vi "4155C Transfer-FPP v2.0.vi"(0 "VISA resource name in":refnum<visa-resource-name>="GPIB0::14::INSTR", 1 "FPP - Source":u32(ring) items=["VSU1  ", "VSU2  "], 2 "Gate":T4={"Gate Start"=0.0, "Gate Stop"=2.0, "Gate Step (linear only)"=1.0, "Gate Compliance"=0.0001, "Gate PComp"=0.0, "Range mode"=0, "Range"=6} {"Range" max=11 scale=0.0..11.0; "Range mode" items=["Auto", "Limited", "Fixed"]; "Gate PComp" min=0.0 max=2.0 format="%^.2e"; "Gate Compliance" min=0.0 max=0.1 format="%^.2e"; "Gate Step (linear only)" min=-100.0 max=100.0 format="%^.4e"; "Gate Stop" min=-100.0 max=100.0 format="%^.4e"; "Gate Start" min=-100.0 max=100.0 format="%^.4e"}, 3 "Drain":T5={"Drain Start"=0.0, "Drain Stop"=2.0, "Drain Compliance"=0.0001, "Drain Step"=1.0, "Drain PComp"=0.0, "Range mode"=0, "Range"=6} {"Range" max=11 scale=0.0..11.0; "Range mode" items=["Auto", "Limited", "Fixed"]; "Drain PComp" min=0.0 max=2.0 format="%^.2e"; "Drain Step" min=-100.0 max=100.0 format="%^.4e"; "Drain Compliance" min=0.0 max=0.1 format="%^.2e"; "Drain Stop" min=-100.0 max=100.0 format="%^.4e"; "Drain Start" min=-100.0 max=100.0 format="%^.4e"}, 4 "FPP - Drain":u32(ring)=1 items=["SMU1  ", "SMU2  ", "SMU3  ", "SMU4  ", "SMU5  ", "SMU6  "], 5 "Timings":T3={"integration time"=0, "Short/Long integration time"=0.00064, "hold time (sec)"=0.0, "delay time (sec)"=0.0, "Step Time (0 disables)"=0.0, "sweep method"=0, "Pulse period"=0.005, "Base voltage"=0.0, "Pulse width"=0.0005} {"Pulse width" min=0.0005 max=0.1 step=0.0001 format="%.4f"; "Base voltage" min=-100.0 max=100.0 format="%^.4e"; "Pulse period" min=0.005 max=1.0 step=0.0001 format="%.4f"; "sweep method" items=["Continuous", "Pulsed"]; "Step Time (0 disables)" min=0.0 format="%.2f"; "delay time (sec)" min=0.0 format="%.4f"; "hold time (sec)" min=0.0 format="%.4f"; "Short/Long integration time" min=0.0 format="%^.0e"; "integration time" scale=0.0..2.0}, 6 "error in (no error)":errorcluster, 8 "FPP - Gate":u32(ring)=2 items=["SMU1  ", "SMU2  ", "SMU3  ", "SMU4  ", "SMU5  ", "SMU6  "], 9 "FPP - Probe 1":u32(ring) items=["SMU1  ", "SMU2  ", "SMU3  ", "SMU4  ", "SMU5  ", "SMU6  "], 10 "sweep mode":u16(ring) items=["Single", "Double"], 11 "FPP - Probe 2":u32(ring)=3 items=["SMU1  ", "SMU2  ", "SMU3  ", "SMU4  ", "SMU5  ", "SMU6  "], 12 "Panel Controls":T2={"Emergency Stop"=refnum, "TransGraph Max"=1e-05, "Text/Graph (text=false)"=FALSE} {"TransGraph Max" format="%.2e"}) -> (16 "VG":dbl[](array[numeric]) format="%.2f", 17 "Outparams":T1={"V2 Start"=0.0, "V2 Step"=0.0, "Number of points"=1} {"V2 Step" format="%.2f"; "V2 Start" format="%^.4e"}, 20 "VISA Resource Name out":refnum<visa-resource-name>, 21 "Vprobe2":dbl[](array[numeric]) format="%.2f", 22 "ID":dbl[](array[numeric]) format="%.2f", 23 "IG":dbl[](array[numeric]) format="%.2f", 25 "Vprobe1":dbl[](array[numeric]) format="%.2f", 26 "error out":errorcluster)   [LabVIEW 2016]
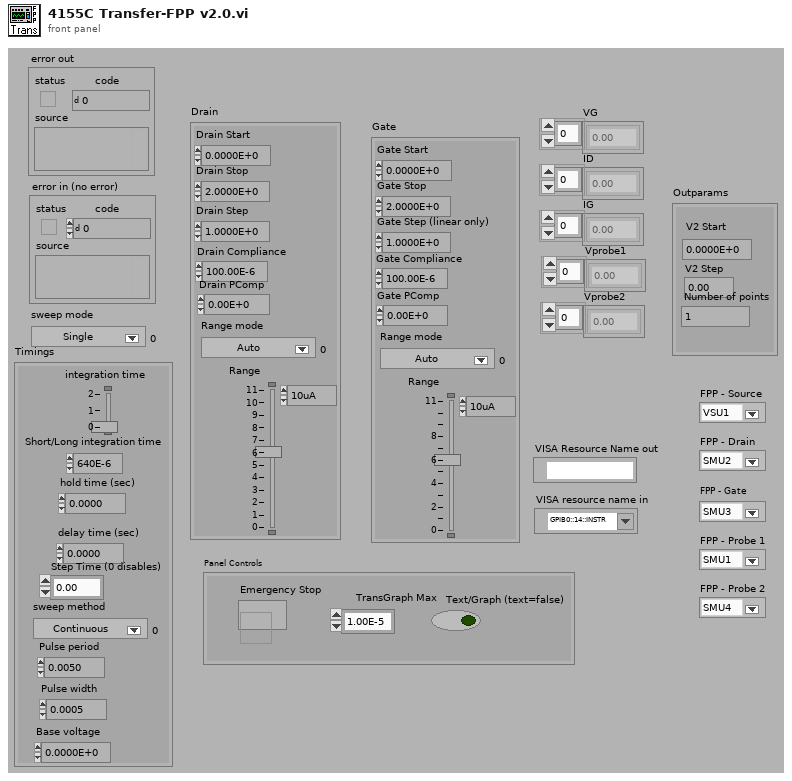
[diagram p1: front panel]
types:
  T1 = cluster{"V2 Start":dbl, "V2 Step":dbl, "Number of points":i32}
  T2 = cluster{"Emergency Stop":refnum<vi>, "TransGraph Max":dbl, "Text/Graph (text=false)":bool}
  T3 = cluster{"integration time":u32, "Short/Long integration time":dbl, "hold time (sec)":dbl, "delay time (sec)":dbl, "Step Time (0 disables)":dbl, "sweep method":u16, "Pulse period":dbl, "Base voltage":dbl, "Pulse width":dbl}
  T4 = cluster{"Gate Start":dbl, "Gate Stop":dbl, "Gate Step (linear only)":dbl, "Gate Compliance":dbl, "Gate PComp":dbl, "Range mode":u16, "Range":u8}
  T5 = cluster{"Drain Start":dbl, "Drain Stop":dbl, "Drain Compliance":dbl, "Drain Step":dbl, "Drain PComp":dbl, "Range mode":u16, "Range":u8}
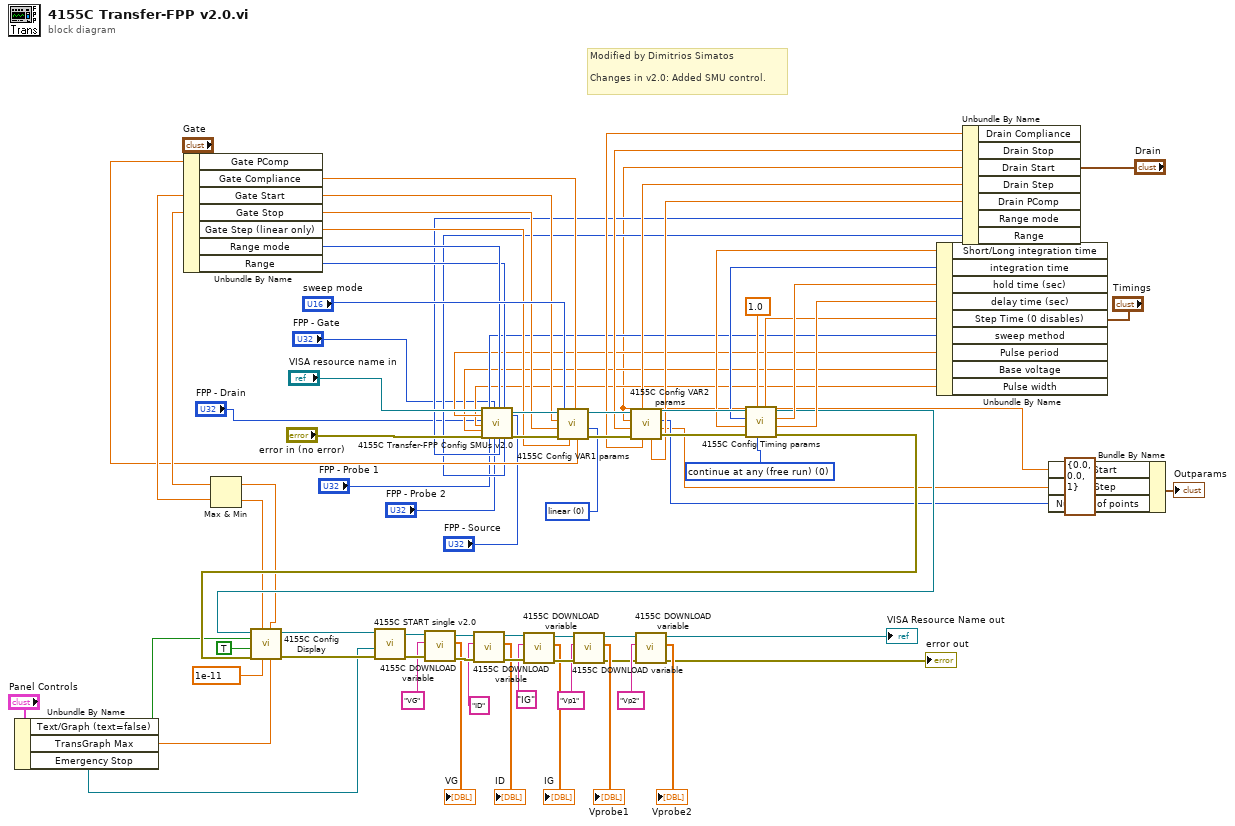
[diagram p0: block diagram]
diagram:
  w65 = u8 0 items=["continue at any (free run)", "stop at any abnorm", "stop at compliance"] ("stop condition (free run:0)")
  w62 = u16 0 items=["linear", "log 10", "log 25", "log 50"] ("sweep spacing (linear: 0)")
  # "Modified by Dimitrios Simatos\n\nChanges in v2.0: Added SMU control."
  n1 = Unbundle By Name("Panel Controls") -> ("Text/Graph (text=false)"=w31:bool, "TransGraph Max"=w32:dbl, "Emergency Stop"=w34:refnum<vi>)
  n2 = Unbundle By Name("Gate") -> ("Gate PComp"=w30:dbl, "Gate Compliance"=w51:dbl, "Gate Start"=w36:dbl, "Gate Stop"=w35:dbl, "Gate Step (linear only)"=w50:dbl, "Range mode"=w28:u16, "Range"=w27:u8)
  n3 = Max & Min(x=w35, y=w36) -> (max(x,y)=w6:dbl, min(x,y)=w7:dbl)
  n4 = Unbundle By Name("Timings") -> ("Short/Long integration time"=w67:dbl, "integration time"=w45:u32, "hold time (sec)"=w46:dbl, "delay time (sec)"=w47:dbl, "Step Time (0 disables)"=w44:dbl, "sweep method"=w24:u16, "Pulse period"=w23:dbl, "Base voltage"=w21:dbl, "Pulse width"=w22:dbl)
  n5 = Unbundle By Name("Drain") -> ("Drain Compliance"=w54:dbl, "Drain Stop"=w53:dbl, "Drain Start"=w16:dbl, "Drain Step"=w52:dbl, "Drain PComp"=w29:dbl, "Range mode"=w26:u16, "Range"=w25:u8)
  n6 = call "4155C Transfer-FPP Config SMUs v2.0.vi"("VISA resource name in"="VISA resource name in", "Pulse period"=w23, "FPP - Drain"="FPP - Drain", "Pulse width"=w22, "Base voltage"=w21, "error in (no error)"="error in (no error)", "sweep method"=w24, "FPP - Probe 1"="FPP - Probe 1", "FPP - Gate"="FPP - Gate", "FPP - Probe 2"="FPP - Probe 2", "Gate mode"=w28, "Source/drain mode"=w26, "Gate Range"=w27, "Source/drain Range"=w25, "FPP - Source"="FPP - Source") -> ("VISA Resource Name out"=w60:refnum<visa-resource-name>, "error out"=w59:errorcluster)  [unwired: 3 in]
  n7 = call "4155C Config VAR1 params.vi"("sweep spacing (linear: 0)"=w62, "power compliance (0 = OFF)"=w30, "compliance"=w51, "step (linear only)"=w50, "sweep mode"="sweep mode", "error in (no error)"=w59, "stop"=w35, "start"=w36, "VISA session"=w60) -> ("error out"=w63:errorcluster, "dup VISA resource name"=w64:refnum<visa-resource-name>)  [unwired: 1 out]
  n8 = call "4155C Config VAR2 params.vi"("power compliance (0 = OFF)"=w29, "compliance"=w54, "step"=w52, "error in (no error)"=w63, "stop"=w53, "start"=w16, "VISA session"=w64) -> ("error out"=w68:errorcluster, "Corrected Step"=w17:dbl, "Number of points"=w18:i32, "dup VISA resource name"=w69:refnum<visa-resource-name>)  [unwired: 1 in]
  n9 = call "4155C Config Timing params.vi"("delay time (sec)"=w47, "hold time (sec)"=w46, "Step Time (0 disables)"=w44, "stop condition (free run:0)"=w65, "wait time parameter"=1.0, "error in (no error)"=w68, "Short/Long integration time"=w67, "integration time"=w45, "VISA session"=w69) -> ("error out"=w38:errorcluster, "dup VISA resource name"=w37:refnum<visa-resource-name>)  [unwired: 1 in]
  n10 = call "4155C Config Display.vi"("Ymax"=w32, "Var1 Stop"=w6, "Ymin"=1e-11, "Var1 Start"=w7, "error in (no error)"=w38, "Logarithmic"=TRUE, "SPA Display"=w31, "VISA session"=w37) -> ("error out"=w39:errorcluster, "dup VISA resource name"=w40:refnum<visa-resource-name>)  [unwired: 2 in]
  n11 = call "4155C START single v2.0.vi"("error in (no error)"=w39, "Emergency Stop"=w34, "VISA resource name in"=w40) -> ("error out"=w80:errorcluster, "VISA Resource Name out"=w81:refnum<visa-resource-name>)  [unwired: 3 in]
  n12 = call "4155C DOWNLOAD variable.vi"("error in (no error)"=w80, "Variable name"="VG", "VISA resource name in"=w81) -> ("error out"=w78:errorcluster, "Output data"=→"VG":dbl[], "VISA Resource Name out"=w77:refnum<visa-resource-name>)  [unwired: 2 in]
  n13 = call "4155C DOWNLOAD variable.vi"("error in (no error)"=w78, "Variable name"="ID", "VISA resource name in"=w77) -> ("error out"=w74:errorcluster, "Output data"=→"ID":dbl[], "VISA Resource Name out"=w75:refnum<visa-resource-name>)  [unwired: 2 in]
  n14 = call "4155C DOWNLOAD variable.vi"("error in (no error)"=w74, "Variable name"="IG", "VISA resource name in"=w75) -> ("error out"=w73:errorcluster, "Output data"=→"IG":dbl[], "VISA Resource Name out"=w72:refnum<visa-resource-name>)  [unwired: 2 in]
  n15 = call "4155C DOWNLOAD variable.vi"("error in (no error)"=w73, "Variable name"="Vp1", "VISA resource name in"=w72) -> ("error out"=w11:errorcluster, "Output data"=→"Vprobe1":dbl[], "VISA Resource Name out"=w12:refnum<visa-resource-name>)  [unwired: 2 in]
  n16 = call "4155C DOWNLOAD variable.vi"("error in (no error)"=w11, "Variable name"="Vp2", "VISA resource name in"=w12) -> ("error out"=→"error out":errorcluster, "Output data"=→"Vprobe2":dbl[], "VISA Resource Name out"=→"VISA Resource Name out":refnum<visa-resource-name>)  [unwired: 2 in]
  n17 = Bundle By Name(cluster=T1 {"V2 Start"=0.0, "V2 Step"=0.0, "Number of points"=1} ("Outparams"), "V2 Start"=w16, "V2 Step"=w17, "Number of points"=w18) -> (→"Outparams":T1)
